vi "log save.vi"(8 "queue out":refnum<queue>, 11 "Instrument Ref":refnum<k24>) -> ()   [LabVIEW 2019, in "SubVI.lvlib"]
uses:
  SubVI.lvlib
  config.ctl
  Instrument.ctl
  lib/QDInstrument.dll
  <vilib>/Utility/file.llb/Write Delimited Spreadsheet (string).vi
panel:
  out "Temperature\nStatus 2":i32(ring) items=["TemperatureUnknown"=0, "Stable"=1, "Tracking"=2, "Near"=5, "Chasing"=6, "Filling"=7, "Standby"=10, "Disabled"=13, "ImpedanceNotFunction"=14, "TempFailure"=15]
  out "Chamber\nStatus 2":i32(ring) items=["ChamberUnknown"=0, "PurgedAndSealed"=1, "VentedAndSealed"=2, "Sealed"=3, "Purging"=4, "Venting"=5, "PreHiVac"=6, "HighVac"=7, "PumpContinuous"=8, "VentContinuous"=9, "ChamberFailure"=15]
  out "Field\nStatus 2":i32(ring) items=["MagnetUnknown"=0, "StablePersistent"=1, "WarmingSwitch"=2, "CoolingSwitch"=3, "StableDriven"=4, "Iterating"=5, "Charging"=6, "Discharging"=7, "CurrentError"=8, "MagnetFailure"=15]
  # "(真是通道1，假是通道2)"
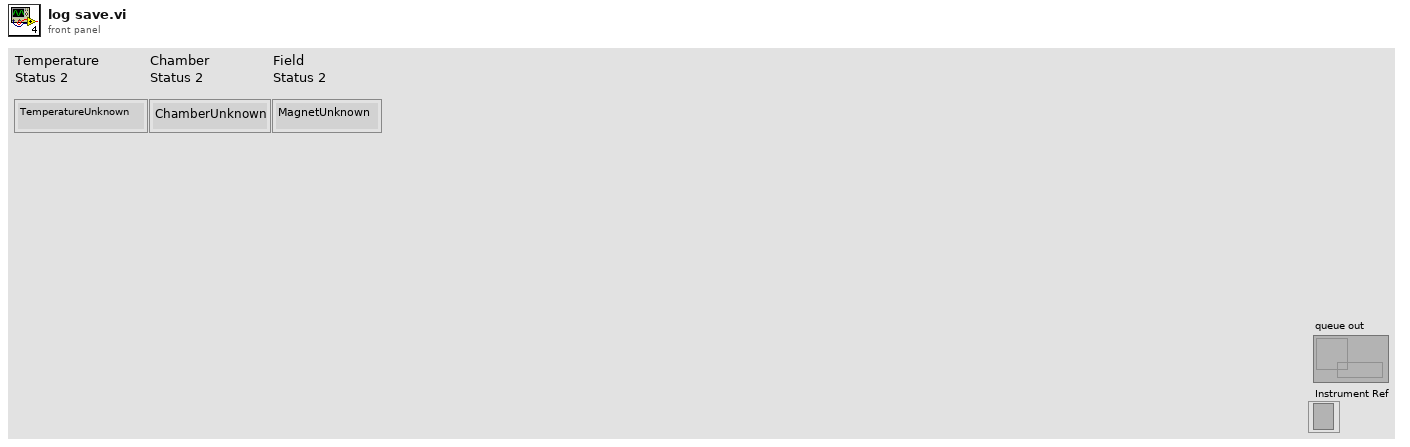
[diagram p1: front panel]
types:
  T1 = typedef "config.ctl" = cluster{"initialize":string, "6221":cluster{"6221 Resource":refnum<visa-resource-name>, "Delta status":bool}, "7001":cluster{"Ch":bool}, "SR830+6221":cluster{"source":u16, "阻抗":dbl, "量程入 4":i32, "量程入 3":i32, "量程入 2":i32, "量程入 1":i32, "电流":dbl, "SR830 2":bool, "SR830 3":bool, "SR830 4":bool, "SR830 1":bool, "VISA 1":refnum<visa-resource-name>, "VISA 2":refnum<visa-resource-name>, "VISA 3":refnum<visa-resource-name>, "VISA 4":refnum<visa-resource-name>, "量程":enum16{"量程每次测量会判定", "量程不变为设定值"}}, "2400":cluster{"2400":bool, "VISA":refnum<visa-resource-name>}, "ch":cluster{"ch str":string, "ch1":bool, "ch2":bool, "布尔":bool}, "error":bool, "数据文件路径":path, "log":cluster{"log路径":path, "log interval":dbl}, "Instrument":T2}
  T2 = typedef "Instrument.ctl" = cluster{"335 Resource":refnum<visa-resource-name>, "Input (0:A)":u16, "Instrument Type":i32, "quantum design":refnum<k24>, "Heater Output (1:1)":u16}
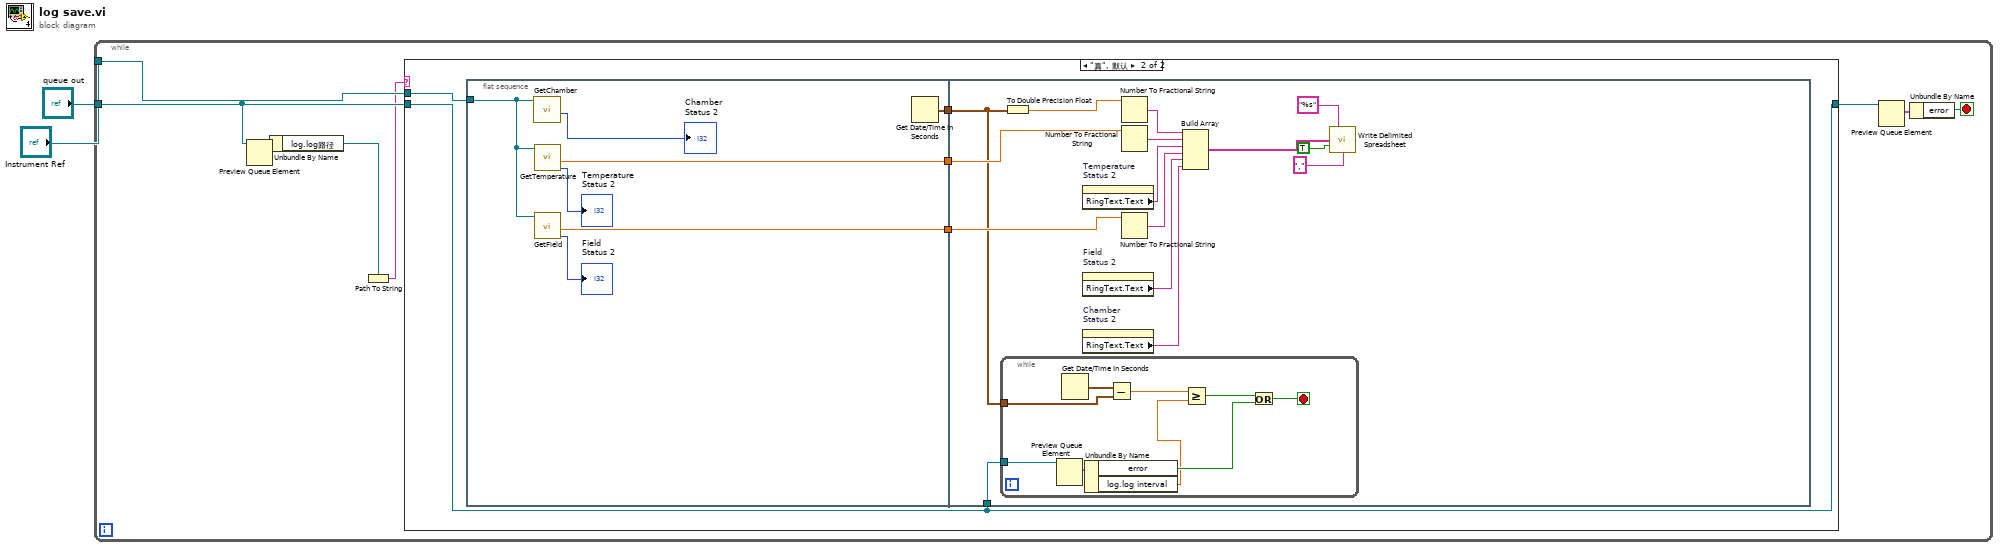
[diagram p0: block diagram]
diagram:
  n1 = while {
    tunnel: "Instrument Ref" -> [w10]
    tunnel: "queue out" -> [w6]
    stop <- w7 stop-if-true
    n2 = Preview Queue Element(queue=w6) -> (element=w5:T1)  [unwired: 2 in, 3 out]
    n3 = Unbundle By Name(w5) -> ("log.log路径"=w4:path)
    n4 = Path To String(path=w4) -> (string=w3:string)
    n5 = case shown="\"真\", 默认" w3 {
      tunnel: w10 -> [_ w13]
      tunnel: w6 -> [w11 w12]
      tunnel: [w11 w12] -> w9
      frame "" {
      }
      frame "真", Default {
        n6 = flat-sequence {
          tunnel: w13 -> [w21]
          tunnel: [w20] -> w15
          tunnel: [w19] -> w16
          tunnel: [w18] -> w14
          tunnel: w16 -> [w30]
          tunnel: w15 -> [w31]
          tunnel: w14 -> [w27]
          tunnel: w12 -> [w26]
          frame #0 {
            n7 = call "GetChamber.vi"("Instrument Ref In"=w21) -> ("Chamber\nStatus"=→"Chamber\nStatus 2":i32)  [unwired: 3 in, 3 out]
            n8 = call "GetTemperature.vi"("Instrument Ref In"=w21) -> ("Temperature\nStatus"=→"Temperature\nStatus 2":i32, "Temperature"=w19:dbl)  [unwired: 4 in, 3 out]
            n9 = call "GetField.vi"("Instrument Ref In"=w21) -> ("Field\nStatus"=→"Field\nStatus 2":i32, "Field"=w20:dbl)  [unwired: 4 in, 3 out]
            n10 = Get Date/Time In Seconds() -> (seconds since 1Jan1904=w18:timestamp)
          }
          frame #1 {
            n11 = while {
              tunnel: w27 -> [w46]
              tunnel: w26 -> [w44]
              stop <- w42 stop-if-true
              n12 = Preview Queue Element(queue=w44) -> (element=w41:T1)  [unwired: 2 in, 3 out]
              n13 = Get Date/Time In Seconds() -> (seconds since 1Jan1904=w47:timestamp)
              n14 = Unbundle By Name(w41) -> ("error"=w40:bool, "log.log interval"=w39:dbl)
              n15 = Subtract(x=w47, y=w46) -> (x-y=w45:dbl)
              n16 = Greater Or Equal?(x=w45, y=w39) -> (x >= y?=w43:bool)
              n17 = Or(x=w43, y=w40) -> (x .or. y?=w42:bool)
            }
            n18 = To Double Precision Float(number=w27) -> (double precision float=w28:dbl)
            n19 = property on="Temperature\nStatus 2" class="Ring (严格)"() -> ("RingText.Text"=w36:string)  [unwired: 2 in, 2 out]
            n20 = property on="Field\nStatus 2" class="Ring (严格)"() -> ("RingText.Text"=w34:string)  [unwired: 2 in, 2 out]
            n21 = property on="Chamber\nStatus 2" class="Ring (严格)"() -> ("RingText.Text"=w33:string)  [unwired: 2 in, 2 out]
            n22 = Number To Fractional String(number=w28) -> (F-format string=w38:string)  [unwired: 3 in]
            n23 = Number To Fractional String(number=w30) -> (F-format string=w37:string)  [unwired: 3 in]
            n24 = Number To Fractional String(number=w31) -> (F-format string=w35:string)  [unwired: 3 in]
            n25 = Build Array(w38, w37, w36, w35, w34, w33) -> (w32:string[])
            n26 = call-poly <vilib>:"Write Delimited Spreadsheet.vi"("format (%s)"="%s", "1D data"=w32, "append to file? (new file:F)"=TRUE, "delimiter (\\t)"="," ("delimiter (\\t)")) -> ()  [unwired: 10 in, 2 out]
          }
        }
      }
    }
    n27 = Preview Queue Element(queue=w9) -> (element=w8:T1)  [unwired: 2 in, 3 out]
    n28 = Unbundle By Name(w8) -> ("error"=w7:bool)
  }
